vi "IRDirection.vi"(11 "BrickReference in":T1) -> (0 "Direction":bool, 3 "BrickReference out":T1)   [LabVIEW 2012, in "BlockParty4150.lvrbt"]
uses:
  BlockParty4150.lvrbt
  <vilib>/NXT/Subs/LVHSConnector.ctl
  <vilib>/NXT/LegoClasses/BrickReference/BrickReference.lvclass
  <vilib>/NXT/Block Support/NXT_ButtonSelector.ctl
  <vilib>/NXT/Dual Mode Library/Display/drawText.vi
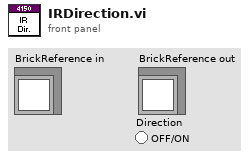
[diagram p1: front panel]
types:
  T1 = typedef "LVHSConnector.ctl" = refnum<class "BrickReference.lvclass">
  T2 = typedef "NXT_ButtonSelector.ctl" = u16
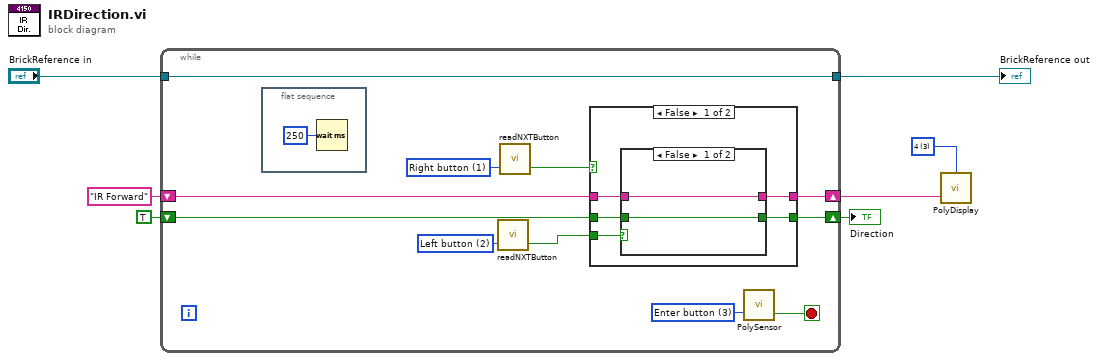
[diagram p0: block diagram]
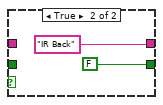
[diagram p2: hidden frame]
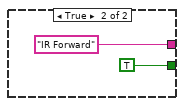
[diagram p3: hidden frame]
diagram:
  w3 = i16 3 items=["1", "2", "3", "4", "5", "6", "7", "8"] ("Line")
  n1 = while {
    tunnel: [w18] -> w6
    tunnel: "BrickReference in" -> [w18]
    shift-right: [w12] -> w4
    shift-left: "IR Forward" -> [w9]
    shift-right: [w10] -> w5
    shift-left: TRUE -> [w8]
    stop <- w16 stop-if-true
    w11 = T2 1 items=["Enter button"=3, "Left button"=2, "Right button"=1] ("Button (Enter button)")
    w13 = T2 2 items=["Enter button"=3, "Left button"=2, "Right button"=1] ("Button (Enter button)")
    w17 = T2 3 items=["Enter button"=3, "Left button"=2, "Right button"=1] ("Button (Enter button)")
    n2 = flat-sequence {
      frame #0 {
        n3 = Wait (ms)(milliseconds to wait=u32 250) -> ()  [unwired: 1 out]
      }
    }
    n4 = call <vilib>:"readNXTButton.vi"("Button (Enter button)"=w13) -> ("Yes/No"=w15:bool)  [unwired: 2 in, 1 out]
    n5 = call <vilib>:"readNXTButton.vi"("Button (Enter button)"=w11) -> ("Yes/No"=w14:bool)  [unwired: 2 in, 1 out]
    n6 = case shown="False" w14 {
      tunnel: w15 -> [w24 _]
      tunnel: [w23 "IR Forward"] -> w12
      tunnel: [w22 TRUE] -> w10
      tunnel: w9 -> [w21 _]
      tunnel: w8 -> [w20 _]
      frame False {
        n7 = case shown="False" w24 {
          tunnel: [w26 "IR Back"] -> w23
          tunnel: [w25 FALSE] -> w22
          tunnel: w21 -> [w26 _]
          tunnel: w20 -> [w25 _]
          frame False {
          }
          frame True {
          }
        }
      }
      frame True {
      }
    }
    n8 = call-poly <vilib>:"PolySensor.vi"("Button (Enter button)"=w17) -> ("Yes/No"=w16:bool)  [unwired: 2 in, 1 out]
  }
  "BrickReference out" <- w6
  "Direction" <- w5
  n9 = call-poly <vilib>:"PolyDisplay.vi"("Text"=w4, "Line"=w3) -> ()  [unwired: 2 in, 1 out]
